vi "SPI Scripting.Create and Place IO Nodes.vi"(4 "Device Icon Name":string[](array[string]), 5 "Device Alias":string, 6 "Block Diagram":refnum<vi>, 7 "Path to IO Node":path=path "D:/Documents/Projects/SPIAPI/IOEngineCode/Initialize Node Resources.vi", 8 "error in":errorcluster, 9 "Path to Analog Node Template":string="IONode\\Analog Input Node x.vi", 10 "Values for Naming":T1={"Bus Number"=1, "Device Number"=1, "Channel Number"=1} {"Channel Number" min=1 step=1; "Device Number" min=1 step=1; "Bus Number" min=1 step=1}, 11 "Virtual Folder":refnum<vi>) -> (0 "error out":errorcluster, 2 "New Copy of IO Node":refnum<vi>, 3 "Path to IO Node":path=path "D:/Documents/Projects/SPIAPI/IOEngineCode/Initialize Node Resources.vi")   [LabVIEW 2014, in "Initialization and IO Node Scripting.lvlib"]
uses:
  Initialization and IO Node Scripting.lvlib
  State Machine/Controls/Values for Naming.ctl
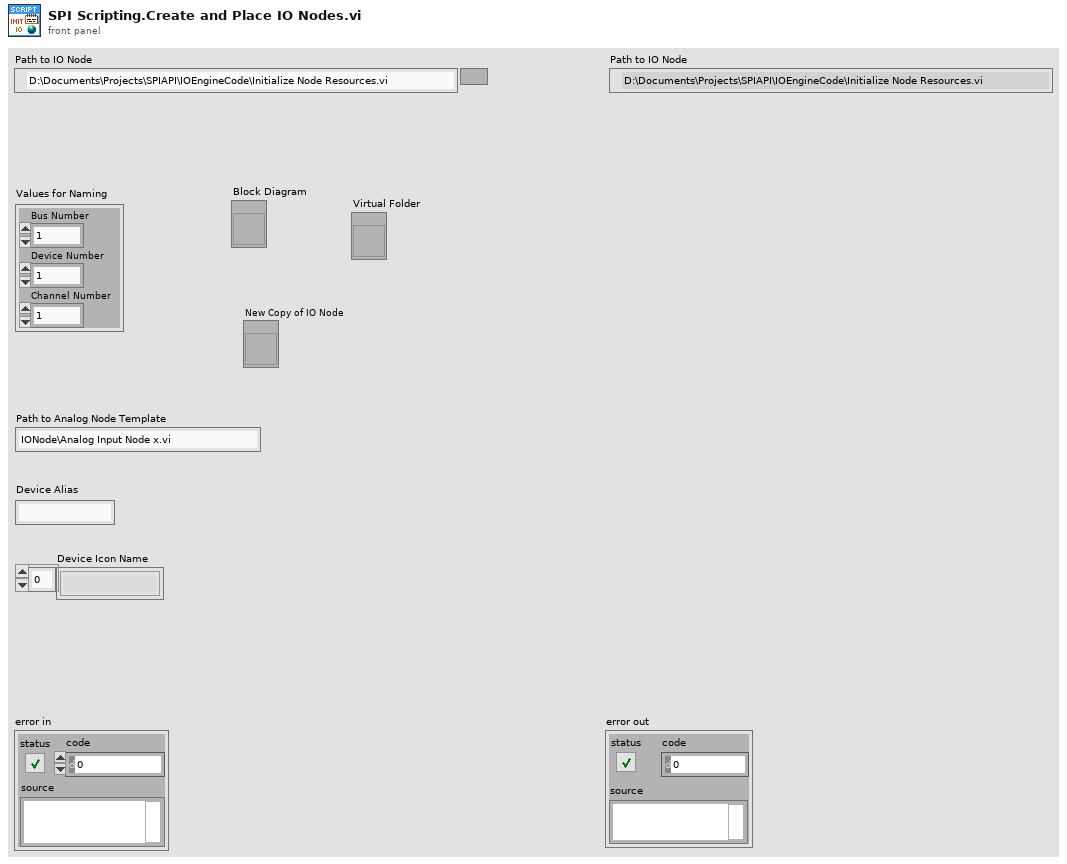
[diagram p1: front panel]
types:
  T1 = typedef "Initialization and IO Node Scripting.lvlib/Values for Naming.ctl" = cluster{"Bus Number":i32, "Device Number":i32, "Channel Number":i32}
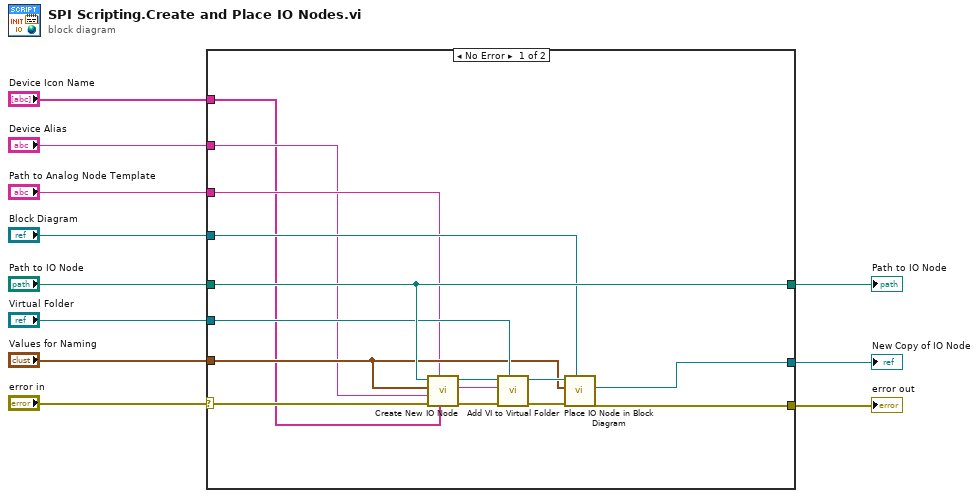
[diagram p0: block diagram]
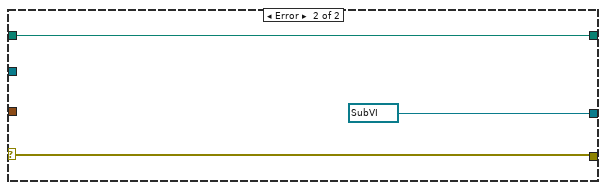
[diagram p2: hidden frame]
diagram:
  n1 = case shown="No Error" "error in" {
    selector: "error in" -> [w17 w29]
    tunnel: "Path to IO Node" -> [w26 w28]
    tunnel: [w18 w29] -> w9
    tunnel: [w26 w28] -> w8
    tunnel: "Block Diagram" -> [w16 _]
    tunnel: [w20 refnum<vi> refnum ("New Copy of IO Node")] -> w6
    tunnel: "Virtual Folder" -> [w19 _]
    tunnel: "Values for Naming" -> [w15 _]
    tunnel: "Path to Analog Node Template" -> [w14 _]
    tunnel: "Device Alias" -> [w13 _]
    tunnel: "Device Icon Name" -> [w12 _]
    frame No Error {
      n2 = call "Create New IO Node.vi"("Device Icon Name"=w12, "Path to Analog Node Template"=w14, "error in"=w17, "Device Alias"=w13, "Values for Naming"=w15, "Path to IO Node"=w26) -> ("error out"=w25:errorcluster, "IO Node Name"=w21:string, "Path to new IO Node"=w24:path)  [unwired: 3 in]
      n3 = call "Add VI to Virtual Folder.vi"("Virtual Folder"=w19, "error in"=w25, "VI Name"=w21, "Path to VI"=w24) -> ("error out"=w22:errorcluster, "Path to VI"=w23:path)  [unwired: 6 in]
      n4 = call "Place IO Node in Block Diagram.vi"("Block Diagram"=w16, "error in"=w22, "Values for Naming"=w15, "Path to New IO Node"=w23) -> ("error out"=w18:errorcluster, "New Copy of IO Node"=w20:refnum<vi>)  [unwired: 6 in]
    }
    frame Error {
    }
  }
  "error out" <- w9
  "Path to IO Node" <- w8
  "New Copy of IO Node" <- w6
